vi "MenuDo.vi"(4 "ModeCol Index":i32=2, 6 "Cell Position":T2, 8 "error in (no error)":errorcluster, 9 "SetList Refs":T1, 10 "ItemTag":string, 11 "MenuDisableCol in":refnum<class "MenuDisableCol.lvclass">) -> (0 "error out":errorcluster, 1 "Table CtlRef Out":refnum<vi>, 2 "Col Array Ref out":refnum<vi>, 3 "MenuDisableCol out":refnum<class "MenuDisableCol.lvclass">, 5 "Update HWI?":bool)   [LabVIEW 2013, in "MenuDisableCol.lvclass"]
doc: "Perform selected shortcut (right-click) menu actions for all columns in general.\nThis VI is read-only w.r.t column data."
uses:
  MenuDisableCol.lvclass
  <vilib>/Utility/miscctls.llb/LVRowAndColumnTypeDef.ctl
  TypeDefs/SetListRefs.ctl
  VariableManagerCodes/VariableManager/VariableManager.lvclass
  TypeDefs/TableHistory.ctl
  TypeDefs/TableArray.ctl
  DeviceVIs/Device/Device.lvclass
  MenuCol/MenuCol.lvclass
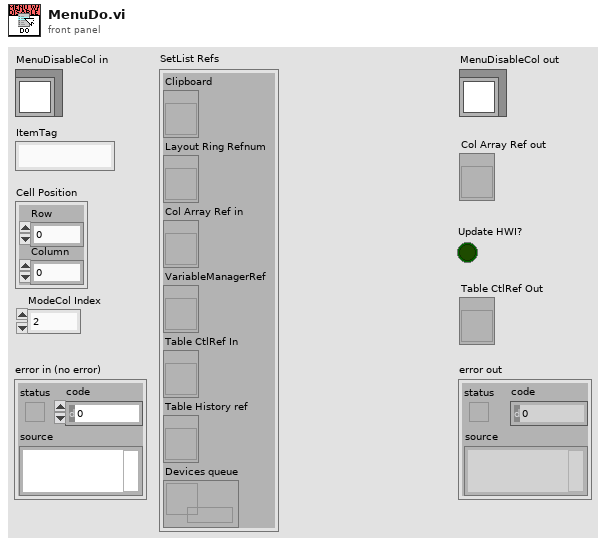
[diagram p1: front panel]
types:
  T1 = typedef "SetListRefs.ctl" = cluster{"Clipboard":refnum<vi>, "Layout Ring Refnum":refnum<vi>, "Col Array Ref in":refnum<vi>, "VariableManagerRef":refnum<vi>, "Table CtlRef In":refnum<vi>, "Table History ref":refnum<vi>, "Devices queue":refnum<queue>}
  T2 = typedef "LVRowAndColumnTypeDef.ctl" = cluster{"Row":i32, "Column":i32}
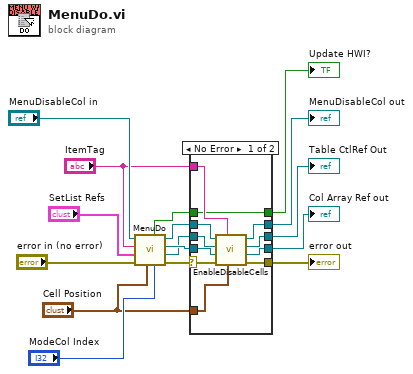
[diagram p0: block diagram]
diagram:
  n1 = call-parent "MenuDo.vi"("ModeCol Index"="ModeCol Index", "Cell Position"="Cell Position", "error in (no error)"="error in (no error)", "SetList Refs"="SetList Refs", "ItemTag"="ItemTag", "MenuCol in"="MenuDisableCol in") -> ("error out"=w13:errorcluster, "Table CtlRef Out"=w5:refnum<vi>, "Col Array Ref out"=w7:refnum<vi>, "MenuCol out"=w12:refnum<class "MenuDisableCol.lvclass">, "Update HWI?"=w9:bool)  [unwired: 1 in]
  n2 = case shown="No Error" w13 {
    selector: w13 -> [w27 w32]
    tunnel: [w25 w32] -> w3
    tunnel: "ItemTag" -> [w20 _]
    tunnel: "Cell Position" -> [w26 _]
    tunnel: [w22 w28] -> w2
    tunnel: w9 -> [w19 w31]
    tunnel: [w19 w31] -> w8
    tunnel: w12 -> [w21 w28]
    tunnel: w7 -> [w17 w30]
    tunnel: w5 -> [w18 w29]
    tunnel: [w23 w29] -> w4
    tunnel: [w24 w30] -> w1
    frame No Error {
      n3 = call-dynamic "EnableDisableCells.vi"("Cell Position"=w26, "Item Name or Tag"=w20, "error in (no error)"=w27, "Col Array Ref in"=w17, "Table CtlRef in"=w18, "MenuDisableCol in"=w21) -> ("error out"=w25:errorcluster, "Col Array Ref out"=w24:refnum<vi>, "Table CtlRef out"=w23:refnum<vi>, "MenuDisableCol out"=w22:refnum<class "MenuDisableCol.lvclass">)  [unwired: 2 in]
    }
    frame Error {
    }
  }
  "error out" <- w3
  "MenuDisableCol out" <- w2
  "Table CtlRef Out" <- w4
  "Col Array Ref out" <- w1
  "Update HWI?" <- w8
